vi "AppendImage.vi"(8 "error in (no error)":errorcluster, 10 "wavename":string, 11 "ITX Commands in":refnum<class "ITX Commands.lvclass">) -> (0 "error out":errorcluster, 3 "ITX Commands out":refnum<class "ITX Commands.lvclass">)   [LabVIEW 2019, in "ITX Commands.lvclass"]
uses:
  ITX Commands.lvclass
panel:
  out "delimited string":string
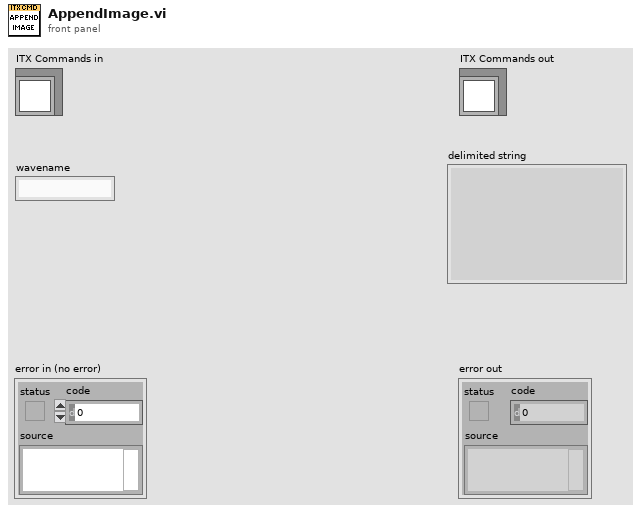
[diagram p1: front panel]
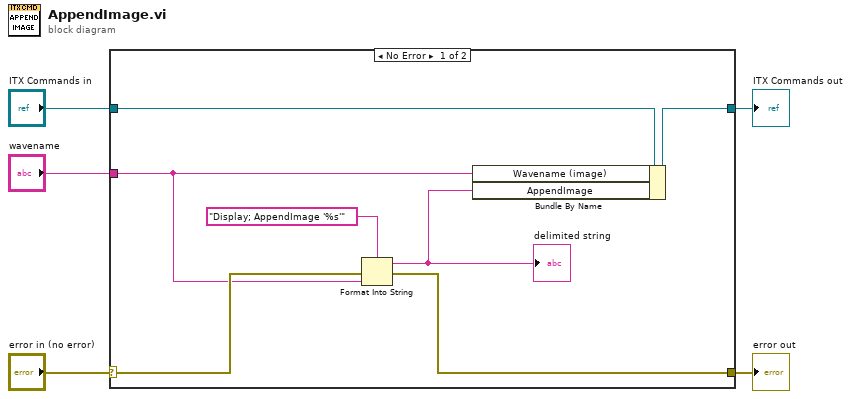
[diagram p0: block diagram]
diagram:
  n1 = case shown="No Error" "error in (no error)" {
    selector: "error in (no error)" -> [w9 w14]
    tunnel: [w7 w14] -> w4
    tunnel: [w11 w13] -> w2
    tunnel: "ITX Commands in" -> [w12 w13]
    tunnel: "wavename" -> [w8 _]
    frame No Error {
      n2 = Format Into String(format string="Display; AppendImage '%s'", error in=w9, w8) -> (resulting string=w6:string, error out=w7:errorcluster)  [unwired: 1 in]
      "delimited string" <- w6
      n3 = Bundle By Name(cluster=w12, "Wavename (image)"=w8, "AppendImage"=w6) -> (w11:refnum<class "ITX Commands.lvclass">)
    }
    frame Error {
    }
  }
  "error out" <- w4
  "ITX Commands out" <- w2
